vi "Get VI Hierarchy Lists.vi"(0 "Top-level VI Paths":path[](array[path]), 11 "error in (no error)":errorcluster) -> (6 "List of VIs":path[](array[path]), 8 "Highest VI Levels":i32[](array[numeric]), 10 "Lowest VI Levels":i32[](array[numeric]), 15 "error out":errorcluster)   [LabVIEW 2010]
doc: "<B>Name:</B>\nGet VI Hierarchy Lists.vi\n<B>References:</B>\nN/A\n<B>Function Description:</B>\nThis VI creates a top-down list of VIs in the hierarchies of the VIs specified by Top-level VI Paths. The list is filtered so that each VI in the hierarchy is listed only once. Since a VI may be located at multiple levels in the hierarchy, two arrays are returned to show the Highest VI Levels and the Lowest VI Levels in the hierarchy. A level of zero (0) represents a top-level VI and the greater the level value, the deeper or lower the level of the VI in the hierarchy.\n\n<B>Inputs:</B>\nTop-level VI Paths: These are the paths of the top-level VIs to include in the generation of the List of VIs and hierarchy levels.\n\nerror in (no error): Standard error in cluster\n\n<B>Outputs:</B>\nList of VIs: This lists VIs in the Top-level VI hierarchy from the top-level to the deepest level.\n\nHighest VI Levels: This array corresponds with the List of VIs to show the highest level in the hierarchy where zero (0) represents the highest possible level.\n\nLowest VI Levels: This array corresponds with the List of VIs to show the lowest level in the hierarchy where greater the numeric value, the lower the hierarchy level.\n\nerror out: Standard error out cluster\n\n<B>Globals:</B>\nN/A\n<B>TestStand Variables:</B>\nN/A\n<B>User Guide:</B>\nN/A\n<B>Control Usage Rules:</B>\nN/A\n<B>VI Interaction:</B>\nN/A\n<B>Occurences:</B>\nN/A\n<B>Devices:</B>\nN/A\n<B>Files:</B>\nN/A\n<B>System Calls:</B>\nN/A\n<B>Keywords:</B>\nhierarchy\n\nAuthor: spcase\nCurrent Revision: 30\nVSS Version: 1\nCopyright 2002 VI Engineering, Inc."
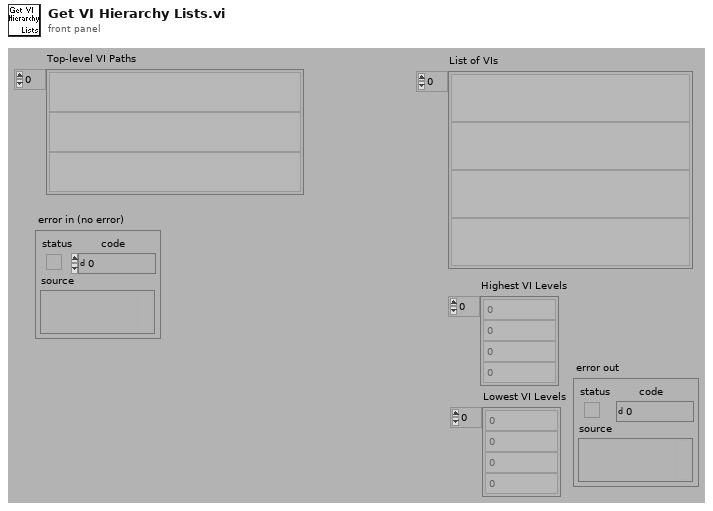
[diagram p1: front panel]
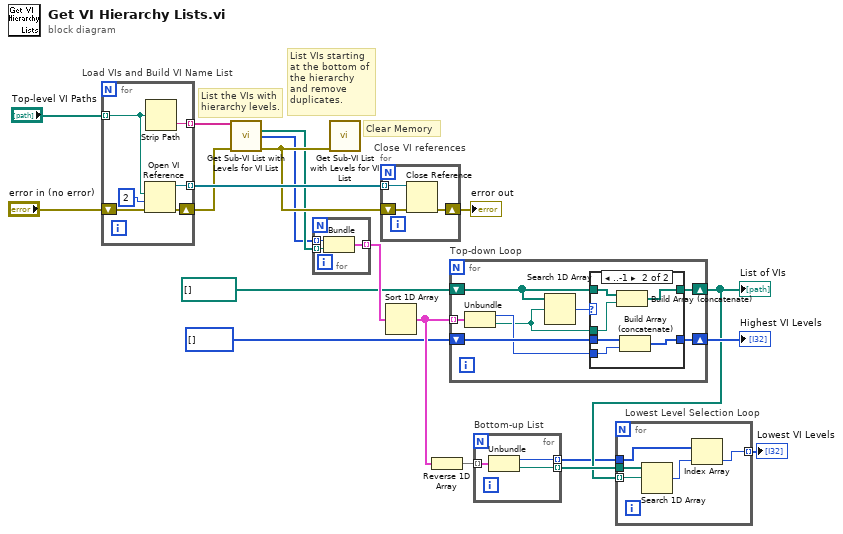
[diagram p0: block diagram]
diagram:
  # "List VIs starting at the bottom of the hierarchy and remove duplicates."
  # "List the VIs with hierarchy levels."
  # "Clear Memory"
  n1 = for "Load VIs and Build VI Name List" {
    tunnel: [w25] -> w16 mode=indexing
    tunnel: [w24] -> w19 mode=indexing
    shift-right: [w22] -> w13
    shift-left: "error in (no error)" -> [w23]
    tunnel: "Top-level VI Paths" -> [w21] mode=indexing
    n2 = Open VI Reference(vi path=w21, options=2, error in (no error)=w23) -> (vi reference=w24:refnum<vi>, error out=w22:errorcluster)  [unwired: 3 in]
    n3 = Strip Path(path=w21) -> (name=w25:string)  [unwired: 1 out]
  }
  n4 = call "Get Sub-VI List with Levels for VI List.vi"("VI List"=w16, "error in (no error)"=w13) -> ("VI Paths"=w10:path[], "VI Levels"=w9:i32[], "error out"=w14:errorcluster)  [unwired: 10 in, 1 out]
  n5 = for {
    tunnel: w9 -> [w28] mode=indexing
    tunnel: w10 -> [w27] mode=indexing
    tunnel: [w26] -> w11 mode=indexing
    n6 = Bundle("Level"=w28, "Path"=w27) -> (w26:cluster{"Level":i32, "Path":path})  [unwired: 1 in]
  }
  n7 = call "Get Sub-VI List with Levels for VI List.vi"("error in (no error)"=w14) -> ()  [unwired: 11 in, 4 out]
  n8 = for "Close VI references" {
    tunnel: w19 -> [w31] mode=indexing
    shift-right: [w29] -> w15
    shift-left: w14 -> [w30]
    n9 = Close Reference(reference=w31, error in (no error)=w30) -> (error out=w29:errorcluster)
  }
  "error out" <- w15
  n10 = Sort 1D Array(array=w11) -> (sorted array=w8:cluster{"Level":i32, "Path":path}[])
  n11 = Reverse 1D Array(array=w8) -> (reversed array=w7:cluster{"Level":i32, "Path":path}[])
  n12 = for "Top-down Loop" {
    shift-right: [w37] -> w3
    shift-left: path[] [] ("Array Constant") -> [w38]
    shift-right: [w35] -> w12
    shift-left: i32[] [] -> [w36]
    tunnel: w8 -> [w34] mode=indexing
    n13 = Unbundle(w34) -> ("Level"=w33:i32, "Path"=w32:path)
    n14 = Search 1D Array(1D array=w38, element=w32) -> (index of element=w39:i32)  [unwired: 1 in]
    n15 = case shown="..-1" w39 {
      tunnel: w38 -> [w41 w47]
      tunnel: [w41 w46] -> w37
      tunnel: w32 -> [_ w45]
      tunnel: w33 -> [_ w42]
      tunnel: w36 -> [w40 w44]
      tunnel: [w40 w43] -> w35
      frame 0.. {
      }
      frame ..-1 {
        n16 = Build Array (concatenate)(w47, w45) -> (w46:path[])
        n17 = Build Array (concatenate)(w44, w42) -> (w43:i32[])
      }
    }
  }
  "List of VIs" <- w3
  "Highest VI Levels" <- w12
  n18 = for "Bottom-up List" {
    tunnel: w7 -> [w50] mode=indexing
    tunnel: [w49] -> w2 mode=indexing
    tunnel: [w48] -> w4 mode=indexing
    n19 = Unbundle(w50) -> ("Level"=w49:i32, "Path"=w48:path)
  }
  n20 = for "Lowest Level Selection Loop" {
    tunnel: w4 -> [w55]
    tunnel: w3 -> [w54] mode=indexing
    tunnel: w2 -> [w52]
    tunnel: [w51] -> w1 mode=indexing
    n21 = Search 1D Array(1D array=w55, element=w54) -> (index of element=w53:i32)  [unwired: 1 in]
    n22 = Index Array(array=w52, index=w53) -> (element=w51:i32)
  }
  "Lowest VI Levels" <- w1
